vi "Benchmark SV Send  LV2012 - NI Verified - 100 Byte - PC - 1Var.vi"() -> ()   [LabVIEW 2015]
panel:
  out "100 byte":i32[][](array[numeric])
  in  "Reset":bool
  out "Tries":u32
  out "Average Delay (ms)":dbl
  out "Delay (ms)":u32
  in  "stop":bool
  # "Overview:  Coding that exemplifies how to benchmark the communication of Shared Variables.\nRequirements: LabVIEW 2012 or compatible\nInstructions:\n1.  Run the \"Benchmark SV Receive LV2012 - NI Verified.vi\"\n2. Run this VI\n3. Watch the amount of time it takes to communicate\n4. Stop both VIs"
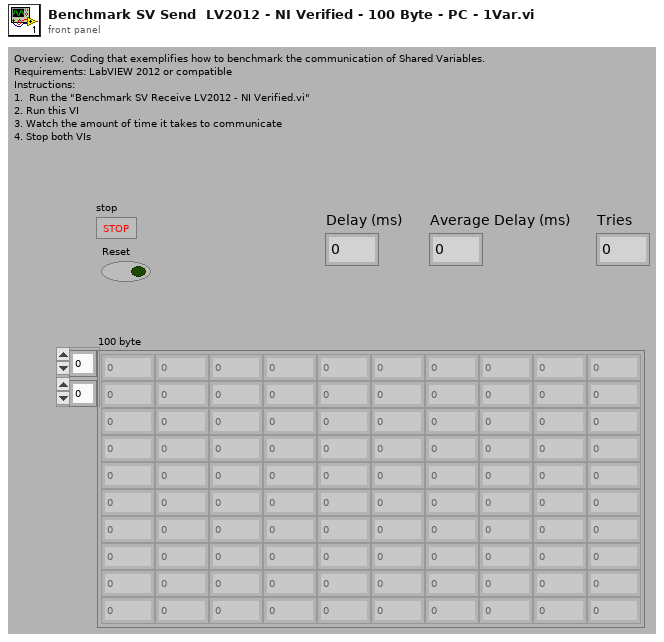
[diagram p1: front panel]
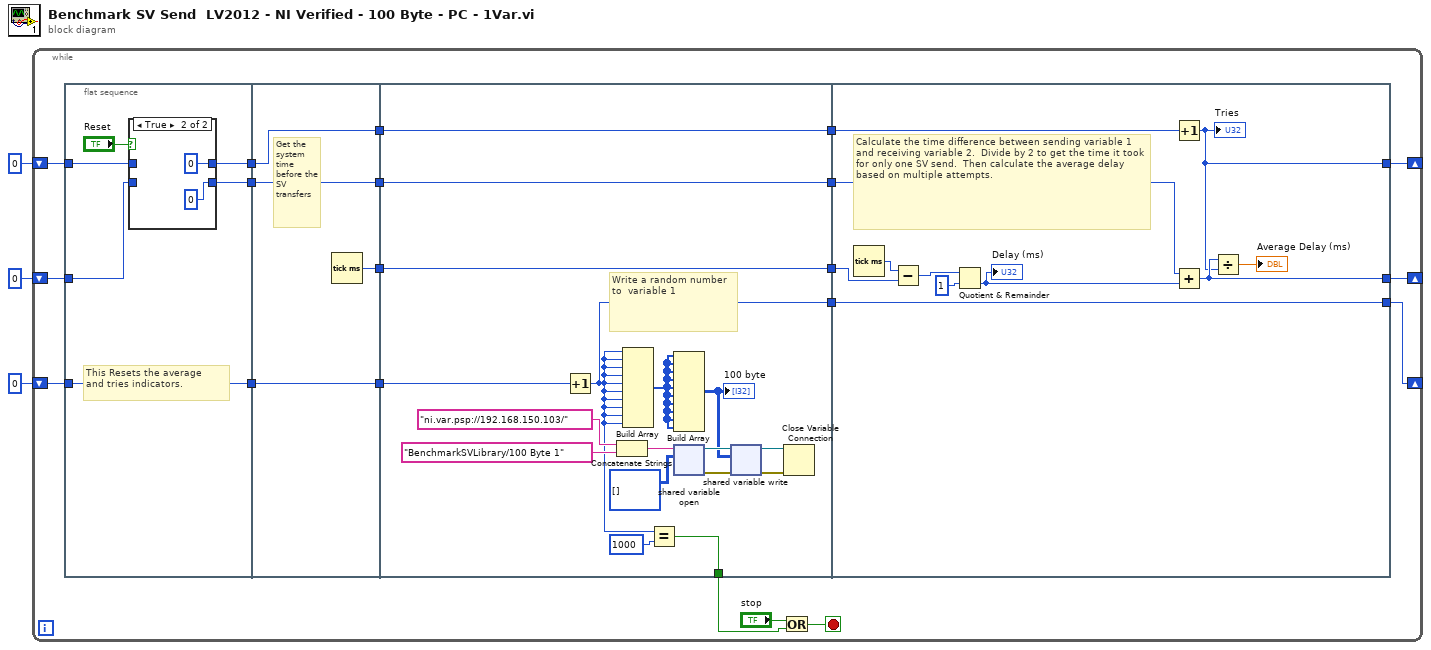
[diagram p0: block diagram]
diagram:
  n1 = while {
    shift-right: [w23] -> _
    shift-left: u32 0 -> [w15]
    shift-right: [w22] -> _
    shift-left: u32 0 -> [w16]
    shift-right: [w11] -> _
    shift-left: 0 -> [w12]
    stop <- w10 stop-if-true
    n2 = flat-sequence {
      tunnel: w15 -> [w29]
      tunnel: [w28] -> w20
      tunnel: [w26] -> w18
      tunnel: w16 -> [w25]
      tunnel: [w24] -> w13
      tunnel: w12 -> [w24]
      tunnel: [w35] -> w21
      tunnel: w20 -> [w37]
      tunnel: [w37] -> w19
      tunnel: w18 -> [w36]
      tunnel: [w36] -> w17
      tunnel: [w34] -> w14
      tunnel: w13 -> [w34]
      tunnel: [w54] -> w7
      tunnel: [w53] -> w6
      tunnel: [w52] -> w5
      tunnel: w21 -> [w54]
      tunnel: w19 -> [w53]
      tunnel: w17 -> [w52]
      tunnel: w14 -> [w44]
      tunnel: [w40] -> w4
      tunnel: [w39] -> w8
      tunnel: w7 -> [w64]
      tunnel: [w57] -> w23
      tunnel: w6 -> [w59]
      tunnel: [w56] -> w22
      tunnel: w5 -> [w63]
      tunnel: w4 -> [w55]
      tunnel: [w55] -> w11
      frame #0 {
        # "This Resets the average \nand tries indicators."
        n3 = case shown="True" "Reset" {
          tunnel: [w31 u32 0] -> w28
          tunnel: w29 -> [w31 _]
          tunnel: [w30 u32 0] -> w26
          tunnel: w25 -> [w30 _]
          frame False {
          }
          frame True {
          }
        }
      }
      frame #1 {
        # "Get the system time before the SV transfers"
        n4 = Tick Count (ms)() -> (millisecond timer value=w35:u32)
      }
      frame #2 {
        # "Write a random number to  variable 1"
        n5 = Increment(x=w44) -> (x+1=w40:i32)
        n6 = Concatenate Strings("ni.var.psp://192.168.150.103/" ("string"), "BenchmarkSVLibrary/100 Byte 1") -> (w47:string)
        n7 = Build Array(w40, w40, w40, w40, w40, w40, w40, w40, w40, w40) -> (w42:i32[])
        n8 = Equal?(x=w40, y=1000) -> (x = y?=w39:bool)
        n9 = Build Array(w42, w42, w42, w42, w42, w42, w42, w42, w42, w42) -> (w41:i32[][])
        "100 byte" <- w41
        n10 = shared-variable-open(w47, i32[][] [] ("appended array")) -> (w51:refnum<k21>, w48:errorcluster)  [unwired: 2 in]
        n11 = shared-variable-write(w51, w48, w41) -> (w49:refnum<k21>, w50:errorcluster)
        n12 = Close Variable Connection(8:w50, 11:w49) -> ()  [unwired: 1 out]
      }
      frame #3 {
        # "Calculate the time difference between sending variable 1 and receiving variable 2.  Divide by 2 to get the time it took for only one SV send.  Then calculate the average delay based on multiple attempts."
        n13 = Tick Count (ms)() -> (millisecond timer value=w65:u32)
        n14 = Subtract(x=w65, y=w64) -> (x-y=w62:u32)
        n15 = Quotient & Remainder(x=w62, y=u32 1) -> (floor(x/y)=w60:u32)  [unwired: 1 out]
        "Delay (ms)" <- w60
        n16 = Increment(x=w63) -> (x+1=w56:u32)
        "Tries" <- w56
        n17 = Add(x=w59, y=w60) -> (x+y=w57:u32)
        n18 = Divide(x=w57, y=w56) -> (x/y=→"Average Delay (ms)":dbl)
      }
    }
    n19 = Or(x="stop", y=w8) -> (x .or. y?=w10:bool)
  }
